vi "Get file.vi"(8 "error in (no error)":errorcluster, 9 "Local path":path, 10 "Remote path":string, 11 "FTP in":refnum<class "FTP.lvclass">) -> (0 "error out":errorcluster, 3 "FTP out":refnum<class "FTP.lvclass">)   [LabVIEW 2015, in "RT Management.lvlib" / "FTP.lvclass"]
uses:
  FTP.lvclass
  FTP.lvclass/FTP.ctl
  File Transfer Behavior/Fix path [scalar].vi
  Get Session.vi
  <vilib>/Utility/error.llb/Trim Whitespace.vi
  File Transfer Behavior/File Transfer Behavior.lvclass
  <vilib>/FTP/NI_FTP.lvlib
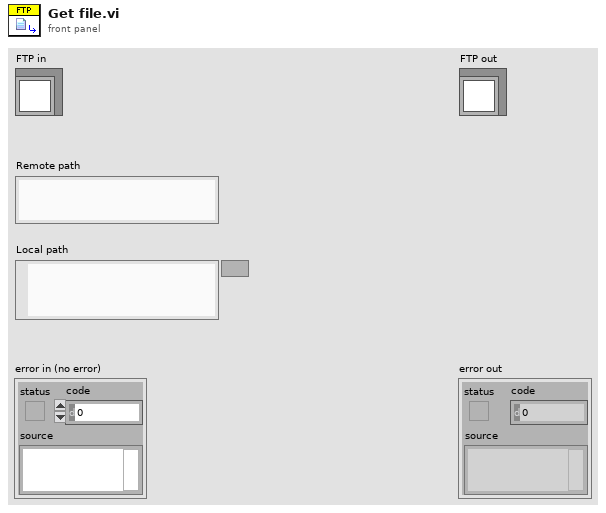
[diagram p1: front panel]
types:
  T1 = cluster{"remote path":string, "local path":path, "binary":bool}
  T2 = typedef "NI_FTP.lvlib/FTP Session.ctl" = refnum<k5>
  T3 = cluster{"remote path":string, "local path":path, "binary":bool}[]
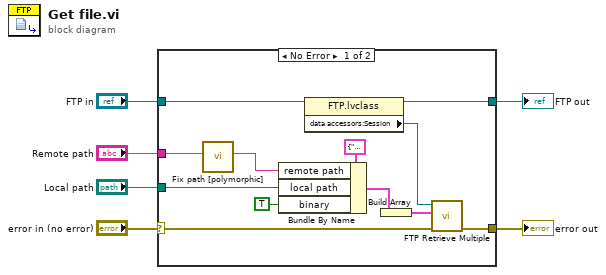
[diagram p0: block diagram]
diagram:
  n1 = case shown="No Error" "error in (no error)" {
    selector: "error in (no error)" -> [w8 w20]
    tunnel: [w15 w20] -> w5
    tunnel: "Remote path" -> [w11 _]
    tunnel: "Local path" -> [w18 _]
    tunnel: "FTP in" -> [w9 w19]
    tunnel: [w7 w19] -> w2
    frame No Error {
      n2 = call-poly "Fix path [polymorphic].vi"("Path in"=w11) -> ("Path out"=w10:string)  [unwired: 8 in, 2 out]
      n3 = Bundle By Name(cluster=T1 {"remote path"="", "local path"=path "", "binary"=FALSE} ("transfer spec"), "remote path"=w10, "local path"=w18, "binary"=TRUE ("active (T)")) -> (w17:T1)
      n4 = property class="FTP.lvclass"(reference=w9) -> (reference out=w7:refnum<class "FTP.lvclass">, "data accessors:Session"=w14:T2)  [unwired: 1 in, 1 out]
      n5 = Build Array(w17) -> (w13:T3)
      n6 = call <vilib>:"FTP Retrieve Multiple.vi"("error in (no error)"=w8, "file specifications"=w13, "ftp session"=w14) -> ("error out"=w15:errorcluster)  [unwired: 2 in, 6 out]
    }
    frame Error {
    }
  }
  "error out" <- w5
  "FTP out" <- w2
